vi "3 seuil.vi"(4 "Seuil":cluster{"Seuil H":dbl, "Seuil B":dbl}, 7 "Temp":dbl(slide) scale=0.0..10.0) -> (0 "Niveaux 1":bool, 1 "Niveaux 2":bool, 2 "Niveaux 3":bool, 3 "Niveaux":i32)   [LabVIEW 2022 SP3]
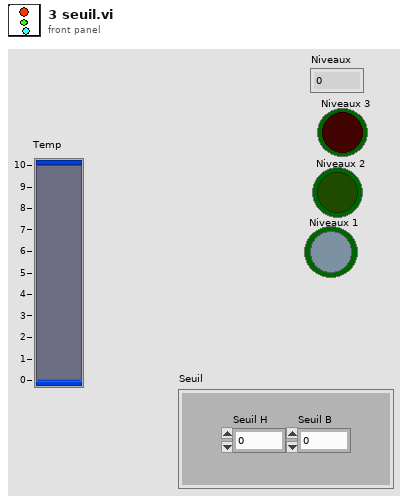
[diagram p1: front panel]
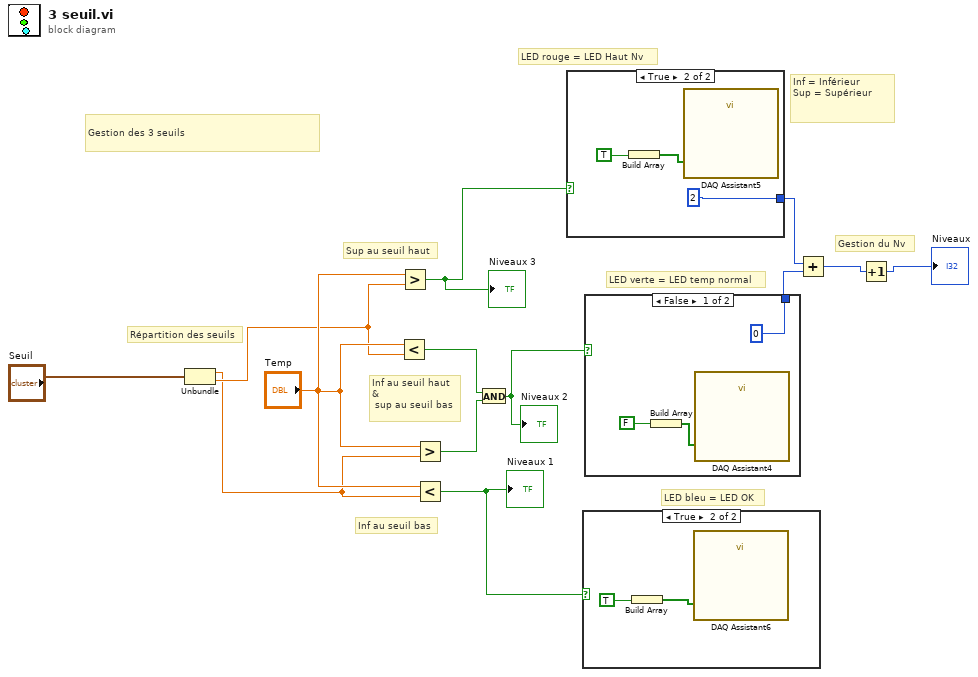
[diagram p0: block diagram]
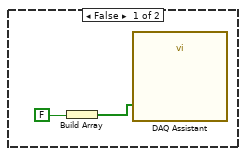
[diagram p2: hidden frame]
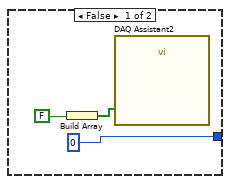
[diagram p3: hidden frame]
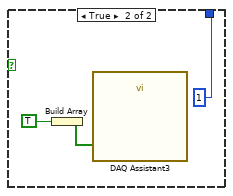
[diagram p4: hidden frame]
diagram:
  # "Inf = Inférieur\nSup = Supérieur"
  # "Gestion des 3 seuils"
  # "Gestion du Nv"
  # "Inf au seuil bas"
  # "Inf au seuil haut \n&\n sup au seuil bas"
  # "Sup au seuil haut"
  # "LED bleu = LED OK"
  # "LED verte = LED temp normal"
  # "LED rouge = LED Haut Nv"
  # "Répartition des seuils"
  n1 = Unbundle "Unbundle"("Seuil") -> ("Seuil H"=w8:dbl, "Seuil B"=w9:dbl)
  n2 = Less?(x="Temp", y=w9) -> (x < y?=w11:bool)
  n3 = Greater?(x="Temp", y=w9) -> (0:w5:bool)
  "Niveaux 3" <- w5
  n4 = Greater?(x="Temp", y=w8) -> (0:w12:bool)
  n5 = Less?(x="Temp", y=w8) -> (x < y?=w4:bool)
  "Niveaux 1" <- w4
  n6 = And(x=w11, y=w12) -> (x .and. y?=w7:bool)
  "Niveaux 2" <- w7
  n7 = case shown="True" w5 {
    tunnel: [0 2] -> w3
    frame False {
      n8 = Build Array(FALSE) -> (w14:bool[])
      n9 = call "DAQ Assistant2"("data"=w14) -> ()  [unwired: 17 in, 2 out]
    }
    frame True {
      n10 = Build Array(TRUE) -> (w17:bool[])
      n11 = call "DAQ Assistant5"("data"=w17) -> ()  [unwired: 17 in, 2 out]
    }
  }
  n12 = case shown="True" w4 {
    frame False {
      n13 = Build Array(FALSE) -> (w20:bool[])
      n14 = call "DAQ Assistant"("data"=w20) -> ()  [unwired: 17 in, 2 out]
    }
    frame True {
      n15 = Build Array(TRUE) -> (w22:bool[])
      n16 = call "DAQ Assistant6"("data"=w22) -> ()  [unwired: 17 in, 2 out]
    }
  }
  n17 = case shown="False" w7 {
    tunnel: [0 1] -> w6
    frame False {
      n18 = Build Array(FALSE) -> (w24:bool[])
      n19 = call "DAQ Assistant4"("data"=w24) -> ()  [unwired: 17 in, 2 out]
    }
    frame True {
      n20 = Build Array(TRUE) -> (w27:bool[])
      n21 = call "DAQ Assistant3"("data"=w27) -> ()  [unwired: 17 in, 2 out]
    }
  }
  n22 = Add(x=w3, y=w6) -> (x+y=w1:i32)
  n23 = Increment(x=w1) -> (x+1=→"Niveaux":i32)
